vi "split_and_dequeue_string.vi"(8 "error in (no error)":errorcluster, 11 "Queue in":refnum<queue>) -> (0 "error out":errorcluster, 1 "argument":string, 2 "state":string, 3 "Queue out":refnum<queue>)   [LabVIEW 2015]
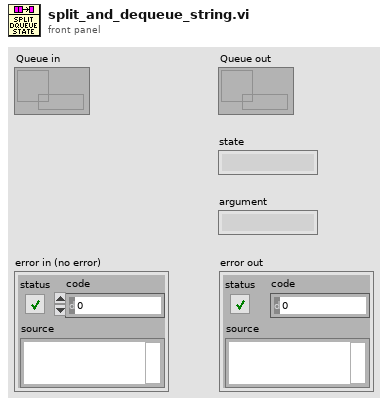
[diagram p1: front panel]
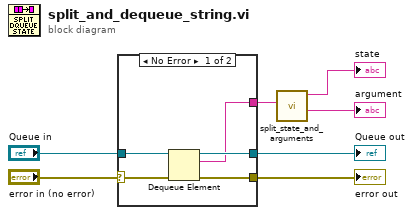
[diagram p0: block diagram]
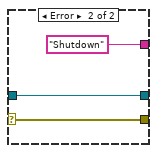
[diagram p2: hidden frame]
diagram:
  n1 = case shown="No Error" "error in (no error)" {
    selector: "error in (no error)" -> [w12 w15]
    tunnel: [w11 w15] -> w2
    tunnel: "Queue in" -> [w10 w14]
    tunnel: [w9 w14] -> w7
    tunnel: [w8 "Shutdown"] -> w6
    frame No Error {
      n2 = Dequeue Element(queue=w10, error in (no error)=w12) -> (queue out=w9:refnum<queue>, element=w8:string, error out=w11:errorcluster)  [unwired: 1 in, 1 out]
    }
    frame Error {
    }
  }
  "Queue out" <- w7
  "error out" <- w2
  n3 = call "split_state_and_arguments.vi"("String"=w6) -> ("Arguments"=→"argument":string, "State"=→"state":string)  [unwired: 9 in]
